vi "Test Lasers.vi"() -> ()   [LabVIEW 2012]
uses:
  <vilib>/Utility/error.llb/DialogType.ctl
  <vilib>/DAQmx/create/channels.llb/DAQmx Create Channel (CO-Pulse Generation-Frequency).vi
  <vilib>/DAQmx/configure/trigger.llb/DAQmx Start Trigger (Digital Edge).vi
  <vilib>/DAQmx/configure/timing.llb/DAQmx Timing (Implicit).vi
  <resource>/objmgr/daqmx.rc
panel:
  in  "stop":bool
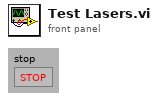
[diagram p1: front panel]
types:
  T1 = typedef "DialogType.ctl" = u16
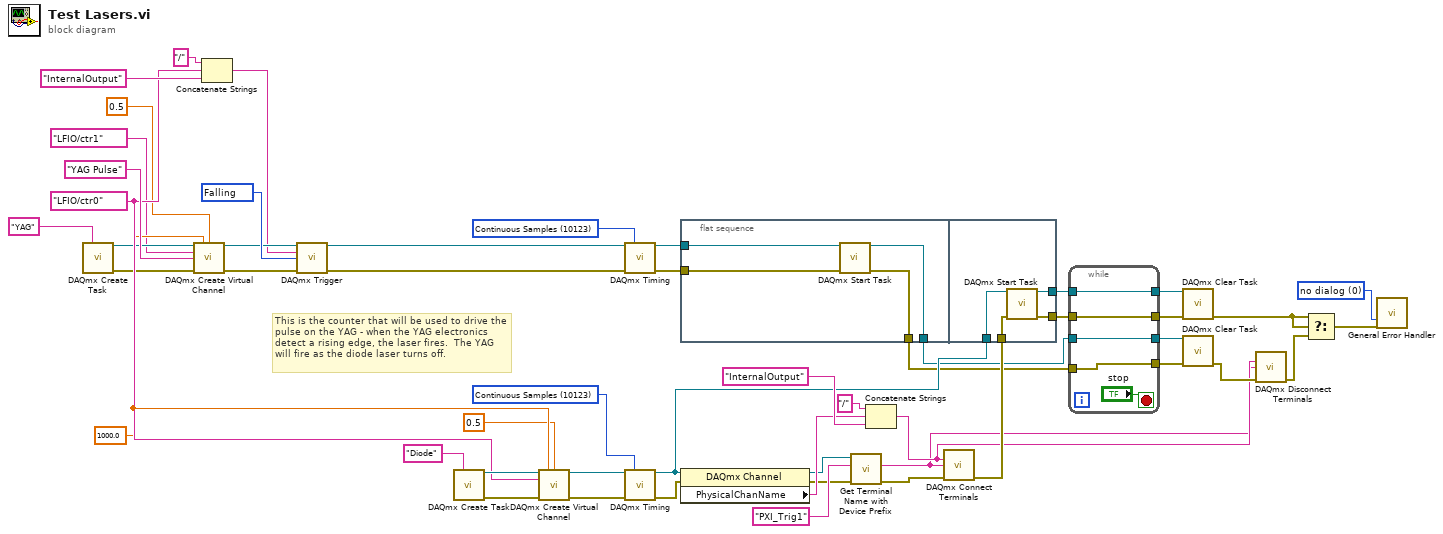
[diagram p0: block diagram]
diagram:
  w25 = T1 0 items=["no dialog", "OK message", "continue or stop message", "OK message + warnings", "continue/stop + warnings"] ("type of dialog (OK msg:1)")
  w32 = 1000.0 ("frequency")
  w37 = tag "LFIO/ctr0" ("counter")
  w43 = 10123 items=["Finite Samples"=10178, "Continuous Samples"=10123, "Hardware Timed Single Point"=12522] ("sample mode")
  w49 = 10171 items=["Rising"=10280, "Falling"=10171] ("edge")
  w51 = 10123 items=["Finite Samples"=10178, "Continuous Samples"=10123, "Hardware Timed Single Point"=12522] ("sample mode")
  # "This is the counter that will be used to drive the pulse on the YAG - when the YAG electronics detect a rising edge, the laser fires.  The YAG will fire as the diode laser turns off."
  n1 = call <vilib>:"DAQmx Create Task.vi"("new task name"="YAG") -> ("task out"=w36:refnum<k21>, "error out"=w35:errorcluster)  [unwired: 13 in]
  n2 = call-poly <vilib>:"DAQmx Create Virtual Channel.vi"("task in"=w36, "frequency"=w32, "duty cycle"=0.5, "counter"=tag "LFIO/ctr1", "name to assign"="YAG Pulse", "error in"=w35) -> ("task out"=w48:refnum<k21>, "error out"=w45:errorcluster)  [unwired: 8 in]
  n3 = Concatenate Strings("/", w37, "InternalOutput" ("string")) -> (w44:string)
  n4 = call-poly <vilib>:"DAQmx Trigger.vi"("task/channels in"=w48, "source"=w44, "edge"=w49, "error in"=w45) -> ("task out"=w42:refnum<k21>, "error out"=w41:errorcluster)  [unwired: 10 in]
  n5 = call <vilib>:"DAQmx Create Task.vi"("new task name"="Diode") -> ("task out"=w39:refnum<k21>, "error out"=w30:errorcluster)  [unwired: 13 in]
  n6 = call-poly <vilib>:"DAQmx Create Virtual Channel.vi"("task in"=w39, "frequency"=w32, "duty cycle"=0.5, "counter"=w37, "error in"=w30) -> ("task out"=w50:refnum<k21>, "error out"=w29:errorcluster)  [unwired: 9 in]
  n7 = call-poly <vilib>:"DAQmx Timing.vi"("task/channels in"=w42, "sample mode"=w43, "error in"=w41) -> ("task out"=w13:refnum<k21>, "error out"=w12:errorcluster)  [unwired: 11 in]
  n8 = call-poly <vilib>:"DAQmx Timing.vi"("task/channels in"=w50, "sample mode"=w51, "error in"=w29) -> ("task out"=w10:refnum<k21>, "error out"=w14:errorcluster)  [unwired: 11 in]
  n9 = flat-sequence {
    tunnel: w13 -> [w55]
    tunnel: w12 -> [w54]
    tunnel: [w53] -> w8
    tunnel: [w52] -> w6
    tunnel: w11 -> [w59]
    tunnel: w10 -> [w58]
    tunnel: [w57] -> w9
    tunnel: [w56] -> w7
    frame #0 {
      n10 = call <vilib>:"DAQmx Start Task.vi"("task/channels in"=w55, "error in"=w54) -> ("task out"=w52:refnum<k21>, "error out"=w53:errorcluster)  [unwired: 12 in]
    }
    frame #1 {
      n11 = call <vilib>:"DAQmx Start Task.vi"("task/channels in"=w58, "error in"=w59) -> ("task out"=w56:refnum<k21>, "error out"=w57:errorcluster)  [unwired: 12 in]
    }
  }
  n12 = property class="DAQmx Channel"(reference=w10, error in=w14) -> (reference out=w16:refnum<k21>, error out=w15:errorcluster, "PhysicalChanName"=w17:tag)
  n13 = call "Get Terminal Name with Device Prefix.vi"("error in (no error)"=w15, "Local Terminal Name"="PXI_Trig1", "task/channels in"=w16) -> ("error out"=w19:errorcluster, "Terminal Name with Device Prefix"=w3:tag)  [unwired: 6 in, 1 out]
  n14 = Concatenate Strings("/", w17, "InternalOutput" ("string")) -> (w4:string)
  n15 = call <vilib>:"DAQmx Connect Terminals.vi"("source terminal"=w4, "destination terminal"=w3, "error in"=w19) -> ("error out"=w11:errorcluster)  [unwired: 12 in]
  n16 = while {
    tunnel: w6 -> [w62]
    tunnel: w7 -> [w63]
    tunnel: [w63] -> w28
    tunnel: [w62] -> w27
    tunnel: w9 -> [w61]
    tunnel: [w61] -> w23
    tunnel: w8 -> [w60]
    tunnel: [w60] -> w22
    stop <- "stop" stop-if-true
  }
  n17 = call <vilib>:"DAQmx Clear Task.vi"("task in"=w28, "error in"=w23) -> ("error out"=w1:errorcluster)  [unwired: 13 in]
  n18 = call <vilib>:"DAQmx Clear Task.vi"("task in"=w27, "error in"=w22) -> ("error out"=w5:errorcluster)  [unwired: 13 in]
  n19 = call <vilib>:"DAQmx Disconnect Terminals.vi"("source terminal"=w4, "destination terminal"=w3, "error in"=w5) -> ("error out"=w2:errorcluster)  [unwired: 12 in]
  n20 = Select(t=w1, s=w1, f=w2) -> (s? t:f=w26:errorcluster)
  n21 = call <vilib>:"General Error Handler.vi"("type of dialog (OK msg:1)"=w25, "error in (no error)"=w26) -> ()  [unwired: 9 in, 5 out]
